vi "sub_cal_vacuum.vi"(11 "vacuum v wf":waveform(dbl) caption="vacuum wf in") -> (3 "vacuum kpa wf":waveform(dbl) caption="vacuum out")   [LabVIEW 2016]
uses:
  <vilib>/Analysis/baseanly.llb/Mean (DBL).vi
  <vilib>/Analysis/NI_AALPro.lvlib
  <vilib>/Analysis/NI_AALBase.lvlib
panel:
  out "vacuum":dbl
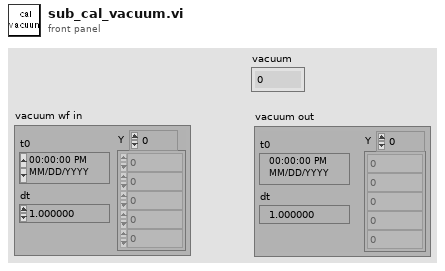
[diagram p1: front panel]
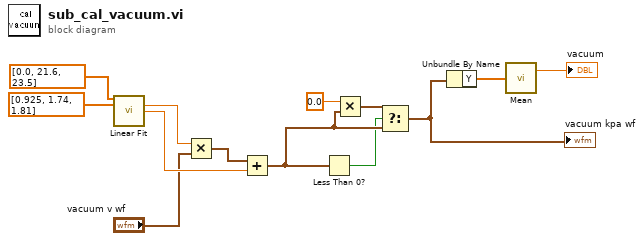
[diagram p0: block diagram]
diagram:
  n1 = call <vilib>:"Linear Fit.vi"("Y"=dbl[] [0.0, 21.6, 23.5] ("X"), "X"=dbl[] [0.925, 1.74, 1.81]) -> ("slope"=w7:dbl, "intercept"=w9:dbl)  [unwired: 9 in, 3 out]
  n2 = Multiply(x=w7, y="vacuum v wf") -> (x*y=w8:waveform(dbl))
  n3 = Add(x=w8, y=w9) -> (x+y=w5:waveform(dbl))
  n4 = Less Than 0?(x=w5) -> (x < 0?=w4:bool)
  n5 = Multiply(x=0.0, y=w5) -> (x*y=w10:waveform(dbl))
  n6 = Select(t=w10, s=w4, f=w5) -> (s? t:f=w1:waveform(dbl))
  "vacuum kpa wf" <- w1
  n7 = Unbundle By Name(w1) -> ("Y"=w6:dbl[])
  n8 = call-poly <vilib>:"Mean.vi"("X"=w6) -> ("mean"=→"vacuum":dbl)  [unwired: 1 out]
